vi "sound_processor.vi"(8 "data in":waveform(dbl), 10 "Target samples per channel":u64=44100, 11 "Volume":dbl(slide) scale=0.0..0.5) -> (0 "data out":waveform(dbl))   [LabVIEW 2022 SP3]
panel:
  out "Array":dbl[](array[numeric])
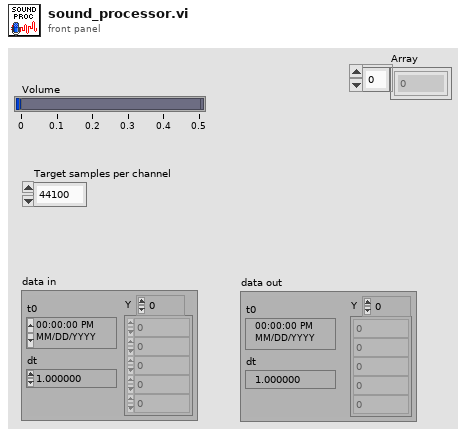
[diagram p1: front panel]
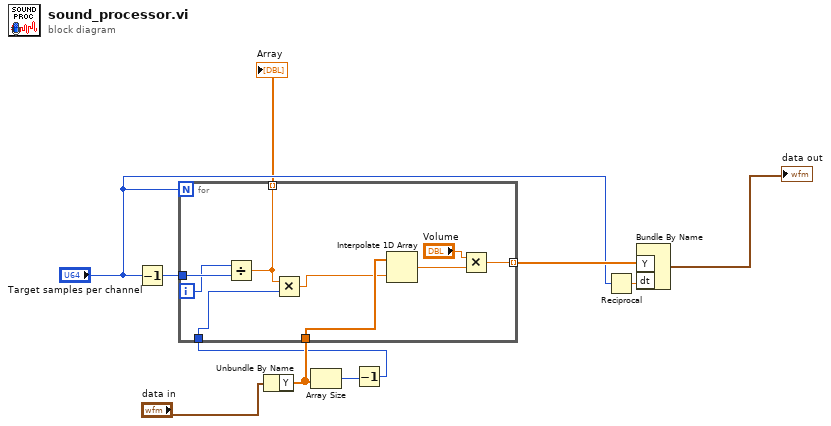
[diagram p0: block diagram]
diagram:
  n1 = Decrement(x="Target samples per channel") -> (x-1=w6:u64)
  n2 = Unbundle By Name("data in") -> ("Y"=w9:dbl[])
  n3 = Array Size(array=w9) -> (size(s)=w2:i32)
  n4 = Decrement(x=w2) -> (x-1=w1:i32)
  n5 = for {
    N: "Target samples per channel" -> [_]
    tunnel: w9 -> [w19]
    tunnel: w1 -> [w12]
    tunnel: [w16] -> w8 mode=indexing
    tunnel: w6 -> [w15]
    tunnel: [w13] -> w3 mode=indexing
    i -> [w14]
    n6 = Divide(x=w14, y=w15) -> (x/y=w13:dbl)
    n7 = Multiply(x=w13, y=w12) -> (x*y=w11:dbl)
    n8 = Interpolate 1D Array(1:w11, 2:w19) -> (0:w17:dbl)
    n9 = Multiply(x="Volume", y=w17) -> (x*y=w16:dbl)
  }
  "Array" <- w3
  n10 = Reciprocal(x="Target samples per channel") -> (1/x=w4:dbl)
  n11 = Bundle By Name("Y"=w8, "dt"=w4) -> (→"data out":waveform(dbl))  [unwired: 1 in]
